vi "Read dsp reset done.vi"(8 "error in (no error)":errorcluster, 11 "niUSRP Rx Core v1 FPGA in":refnum<class "niUSRP Rx Core v1 FPGA.lvclass">=refnum) -> (0 "error out":errorcluster, 2 "dsp reset done":refnum<k21>, 3 "niUSRP Rx Core v1 FPGA out":refnum<class "niUSRP Rx Core v1 FPGA.lvclass">)   [LabVIEW 2023]
uses:
  <instrlib>/niUSRP/Reference FPGA/Rx Core/niUSRP Rx Core v1 FPGA.lvclass
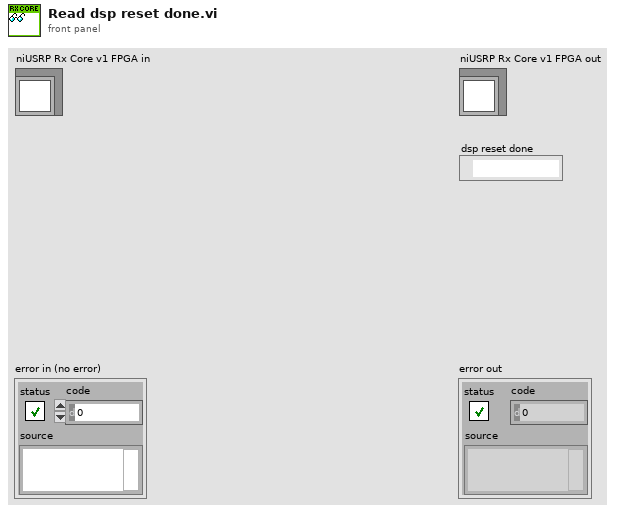
[diagram p1: front panel]
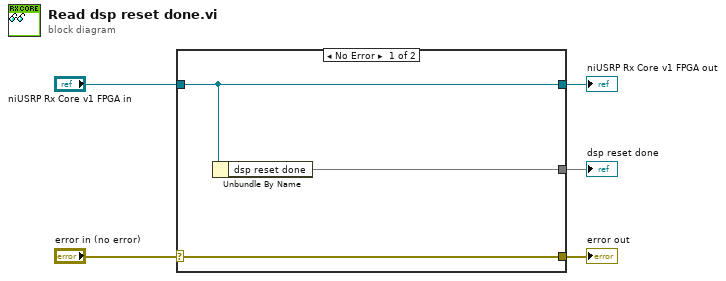
[diagram p0: block diagram]
diagram:
  n1 = case shown="No Error" "error in (no error)" {
    selector: "error in (no error)" -> [w8 w9]
    tunnel: [w8 w9] -> w4
    tunnel: [w7 w10] -> w2
    tunnel: "niUSRP Rx Core v1 FPGA in" -> [w7 w10]
    tunnel: [w6 _] -> w1
    frame No Error {
      n2 = Unbundle By Name(w7) -> ("dsp reset done"=w6)
    }
    frame Error {
    }
  }
  "error out" <- w4
  "niUSRP Rx Core v1 FPGA out" <- w2
  "dsp reset done" <- w1
